vi "3.3-Lidar Filter Ground Plane.vi"(2 "Angle Array":sgl[](array[numeric]), 3 "Magnitude Array":sgl[](array[numeric])) -> (0 "Angle Array":sgl[](array[numeric]), 1 "Magnitude Array":sgl[](array[numeric]))   [LabVIEW 2010]
panel:
  in  "Ground Threshold (mm)":sgl=10.0
  out "Ground Polar Magnitude":dbl
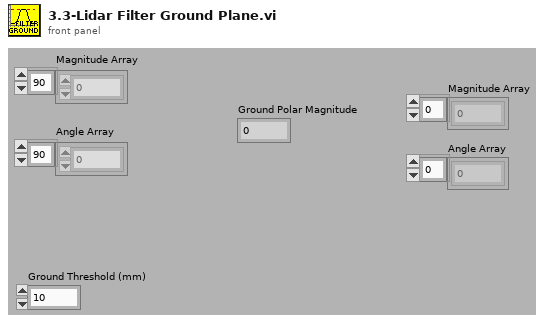
[diagram p1: front panel]
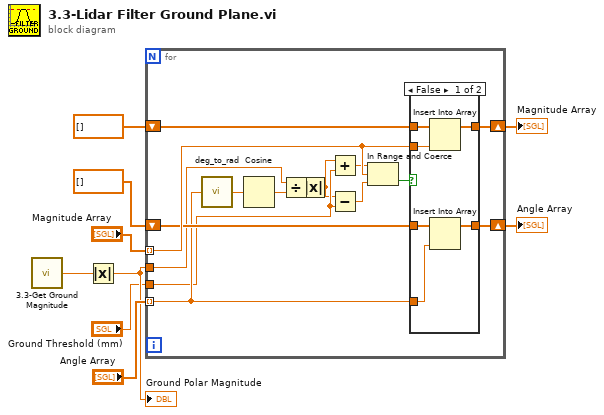
[diagram p0: block diagram]
diagram:
  n1 = call "3.3-Get Ground Magnitude.vi"() -> ("Numeric"=w7:dbl)  [unwired: 1 in]
  n2 = Absolute Value(x=w7) -> (abs(x)=w2:dbl)
  "Ground Polar Magnitude" <- w2
  n3 = for {
    tunnel: "Angle Array" -> [w17] mode=indexing
    tunnel: "Magnitude Array" -> [w23] mode=indexing
    shift-right: [w21] -> w3
    shift-left: sgl[] [] -> [w22]
    shift-right: [w19] -> w4
    shift-left: sgl[] [] -> [w20]
    tunnel: w2 -> [w11]
    tunnel: "Ground Threshold (mm)" -> [w14]
    n4 = call "deg_to_rad.vi"("Degrees"=w17) -> ("Radians"=w18:dbl)
    n5 = Cosine(x=w18) -> (cos(x)=w12:dbl)
    n6 = Divide(x=w11, y=w12) -> (x/y=w15:dbl)
    n7 = Absolute Value(x=w15) -> (abs(x)=w10:dbl)
    n8 = Add(x=w10, y=w14) -> (x+y=w13:dbl)
    n9 = Subtract(x=w10, y=w14) -> (x-y=w16:dbl)
    n10 = In Range and Coerce(upper limit=w13, x=w23, lower limit=w16) -> (In Range?=w24:bool)  [unwired: 1 out]
    n11 = case shown="False" w24 {
      tunnel: w23 -> [w29 _]
      tunnel: w17 -> [w27 _]
      tunnel: w22 -> [w30 w32]
      tunnel: [w28 w32] -> w21
      tunnel: w20 -> [w26 w31]
      tunnel: [w25 w31] -> w19
      frame False {
        n12 = Insert Into Array(array=w30, new element=w29) -> (w28:sgl[])  [unwired: 1 in]
        n13 = Insert Into Array(array=w26, new element=w27) -> (w25:sgl[])  [unwired: 1 in]
      }
      frame True {
      }
    }
  }
  "Angle Array" <- w4
  "Magnitude Array" <- w3
